vi "Create simplified GUI element.vi"(8 "error in (no error)":errorcluster, 10 "Index":i32, 11 "Schedule Block in":refnum<class "Schedule Block.lvclass">) -> (0 "error out":errorcluster, 2 "Simple GUI Element":T1={"Bcg Color"=16777225, "Index"=0, "No. of runs"=0, "Script name"="", "FPGA name"="", "Parameters"="", "Repetitions"=0}, 3 "Schedule Block out":refnum<class "Schedule Block.lvclass">)   [LabVIEW 2020, in "Run Utilities.lvlib" / "Schedule Block.lvclass"]
doc: "Create a GUI element for this SBlock"
uses:
  Schedule Block.lvclass
  Schedule Block - simplified GUI.ctl
  Schedule Block.lvclass/Schedule Block.ctl
  Schedule/Schedule.lvclass
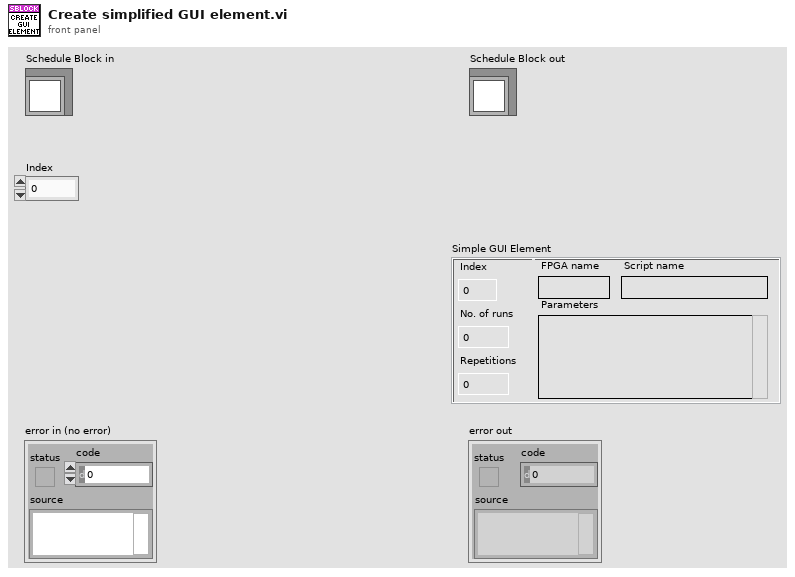
[diagram p1: front panel]
types:
  T1 = typedef "Run Utilities.lvlib/Schedule Block.lvclass/Schedule Block - simplified GUI.ctl" = cluster{"Bcg Color":u32, "Index":i32, "No. of runs":i32, "Script name":string, "FPGA name":string, "Parameters":string, "Repetitions":i32}
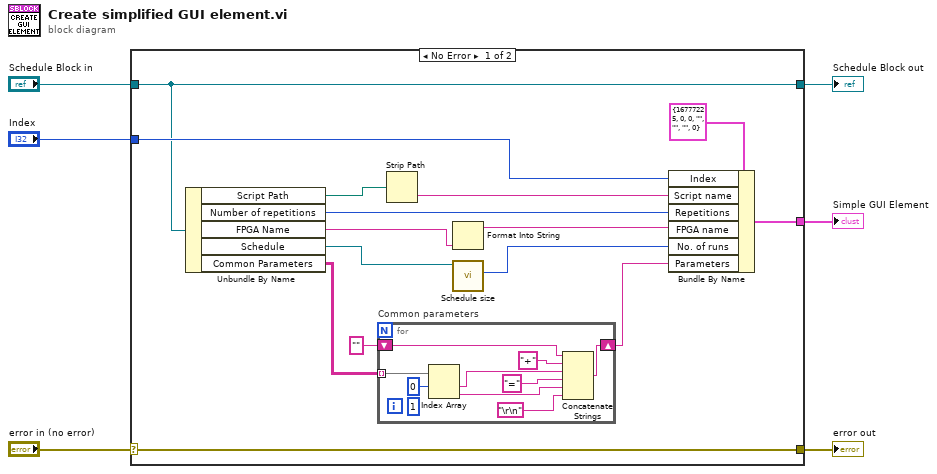
[diagram p0: block diagram]
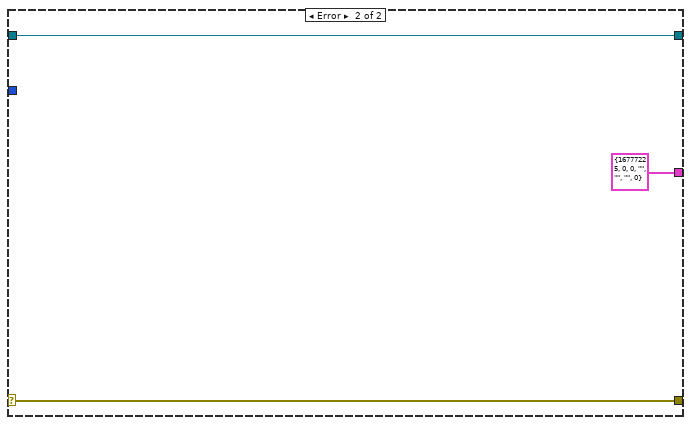
[diagram p2: hidden frame]
diagram:
  n1 = case shown="No Error" "error in (no error)" {
    selector: "error in (no error)" -> [w21 w33]
    tunnel: [w21 w33] -> w5
    tunnel: [w13 w32] -> w3
    tunnel: "Schedule Block in" -> [w13 w32]
    tunnel: [w12 T1 {"Bcg Color"=16777225, "Index"=0, "No. of runs"=0, "Script name"="", "FPGA name"="", "Parameters"="", "Repetitions"=0} ("Cluster")] -> w2
    tunnel: "Index" -> [w16 _]
    frame No Error {
      n2 = Unbundle By Name(w13) -> ("Script Path"=w20:path, "Number of repetitions"=w17:u16, "FPGA Name"=w15:string, "Schedule"=w11:refnum<class "Schedule.lvclass">, "Common Parameters"=w8:string[][])
      n3 = for "Common parameters" {
        tunnel: w8 -> [w25] mode=indexing
        shift-right: [w27] -> w7
        shift-left: "" -> [w26]
        (unwired) 1 ("index")
        n4 = Index Array(array=w25, index #1=0 ("index")) -> (element #1=w24:string, element #2=w23:string)  [unwired: 1 in]
        n5 = Concatenate Strings(w26, "+" ("string"), w24, "=" ("string"), w23, "\r\n") -> (w27:string)
      }
      n6 = Strip Path(path=w20) -> (name=w18:string)  [unwired: 1 out]
      n7 = Format Into String(w15) -> (resulting string=w14:string)  [unwired: 3 in, 1 out]
      n8 = call-dynamic "Schedule size.vi"("Schedule in"=w11) -> ("Size"=w10:i32)  [unwired: 8 in, 2 out]
      n9 = Bundle By Name(cluster=T1 {"Bcg Color"=16777225, "Index"=0, "No. of runs"=0, "Script name"="", "FPGA name"="", "Parameters"="", "Repetitions"=0} ("Cluster"), "Index"=w16, "Script name"=w18, "Repetitions"=w17, "FPGA name"=w14, "No. of runs"=w10, "Parameters"=w7) -> (w12:T1)
    }
    frame Error {
    }
  }
  "error out" <- w5
  "Schedule Block out" <- w3
  "Simple GUI Element" <- w2
